vi "UserConsole.vi"(8 "error in (no error)":errorcluster) -> (0 "error out":errorcluster)   [LabVIEW 2013, in "UserConsole.lvlib"]
doc: "User Console simulates to Keypad,Transactions and Card Insertion."
uses:
  UserConsole.lvlib
  PrivateControls/Keypad.ctl
  PrivateControls/Transactions.ctl
  PrivateControls/UserConsole_QueueDriver.ctl
  MainVI/TopLevelController/ToplevelControllerLibrary.lvlib
panel:
  in  "Transactions":T1
  in  "Keypad":T2
  in  "Card Reader":bool
  # "User Console simulates to Keypad,Transactions and Card Insertion."
  # "[Covers: UI1]"
  # "[Covers: UI2C]"
  # "[Covers: UI2B]"
  # "[Covers: UI2]"
  # "[Covers: UI2A]"
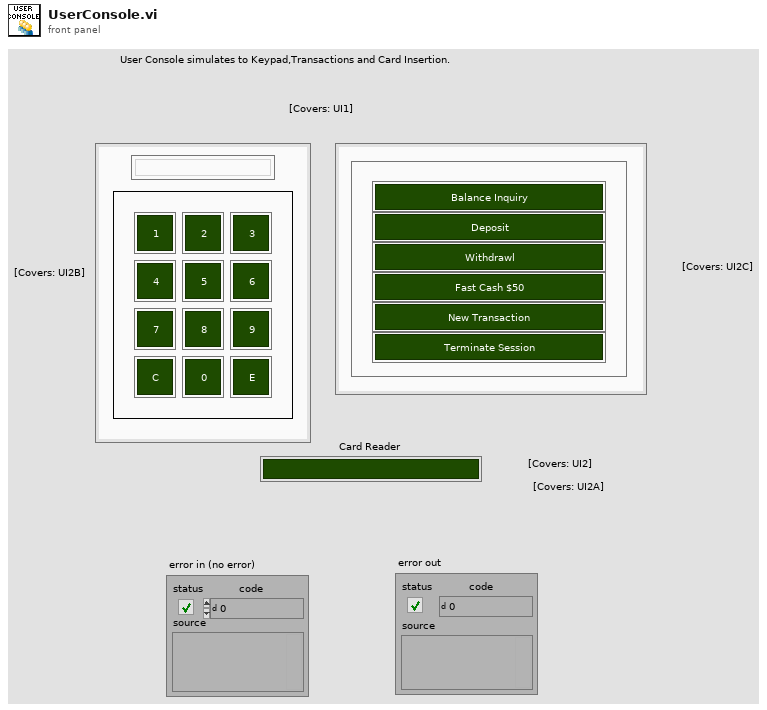
[diagram p1: front panel]
types:
  T1 = typedef "UserConsole.lvlib/Transactions.ctl" = cluster{"xaction":bool, "xaction 2":bool, "xaction 3":bool, "xaction 4":bool, "xaction 5":bool, "xaction 6":bool}
  T2 = typedef "UserConsole.lvlib/Keypad.ctl" = cluster{"Key":bool, "Key 2":bool, "Key 3":bool, "Key 4":bool, "Key 5":bool, "Key 6":bool, "Key 7":bool, "Key 8":bool, "Key 9":bool, "Key 10":bool, "Key 11":bool, "Key 12":bool, "Knumber":string}
  T3 = typedef "UserConsole.lvlib/UserConsole_QueueDriver.ctl" = enum16{"Default Case", "Init", "Enqueue", "Dequeue", "ReleaseQueue", "Exit"}
  T4 = enum16{"Create Event", "Generate Event", "Destroy Event"}
  T5 = enum16{"Init", "Enqueue", "Dequeue", "ReleaseQueue", "Exit"}
  T6 = typedef "UserConsole.lvlib/DataCluster.ctl" = cluster{"Card Reader":bool, "Keypad":cluster{"Key":bool, "Key 2":bool, "Key 3":bool, "Key 4":bool, "Key 5":bool, "Key 6":bool, "Key 7":bool, "Key 8":bool, "Key 9":bool, "Key 10":bool, "Key 11":bool, "Key 12":bool, "Knumber":string}, "Transactions":cluster{"xaction":bool, "xaction 2":bool, "xaction 3":bool, "xaction 4":bool, "xaction 5":bool, "xaction 6":bool}}
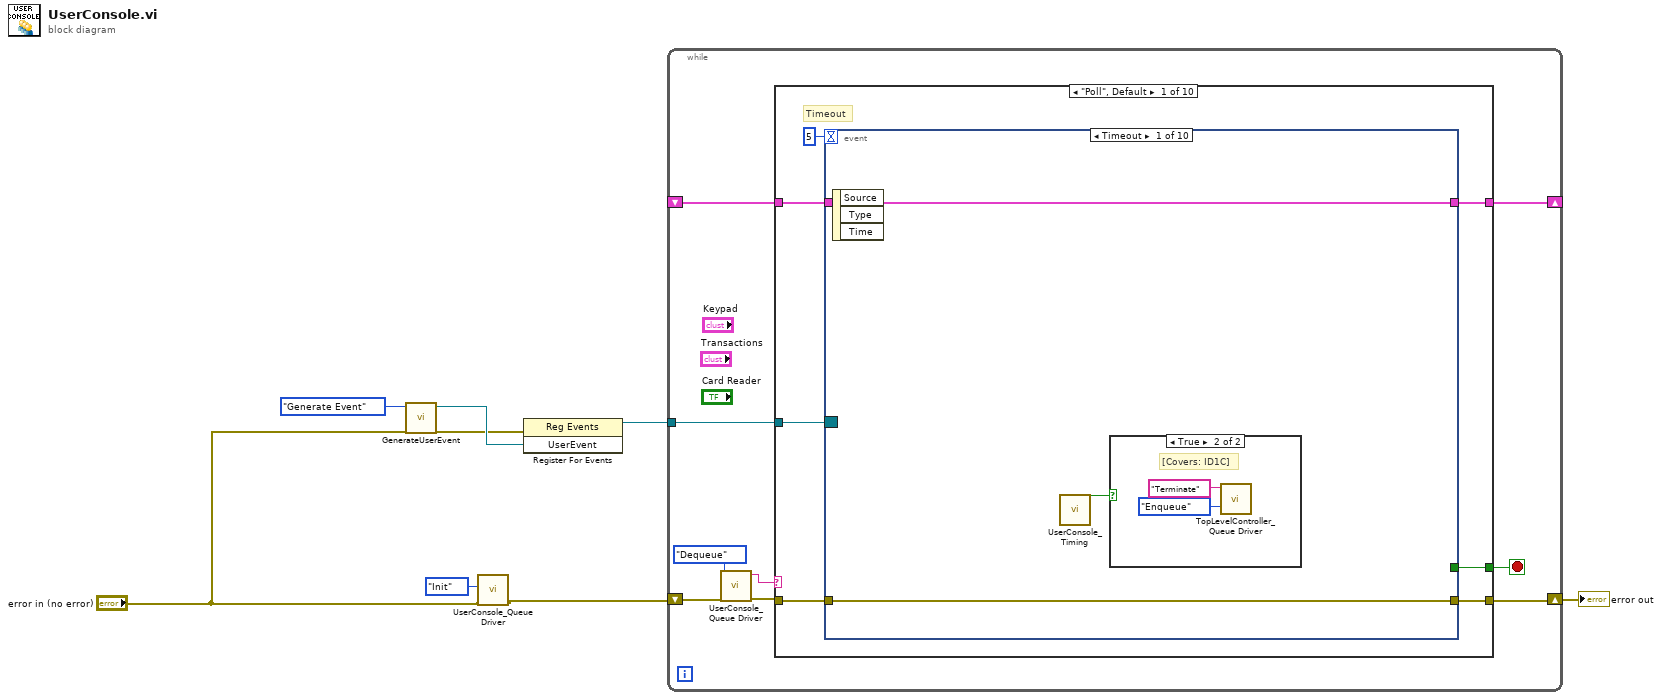
[diagram p0: block diagram]
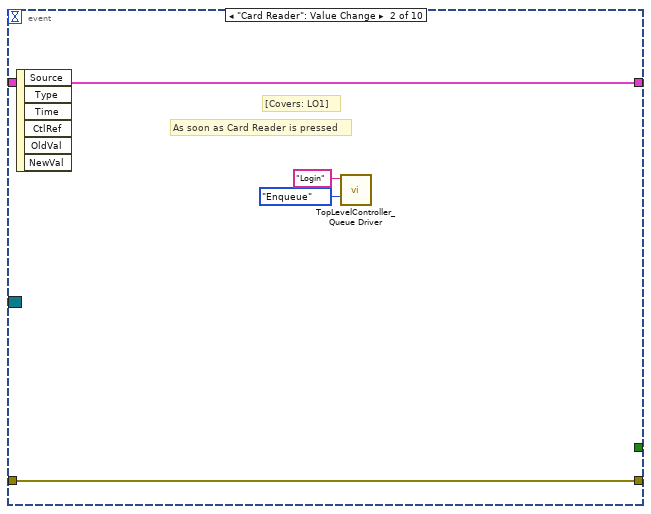
[diagram p3: hidden frame]
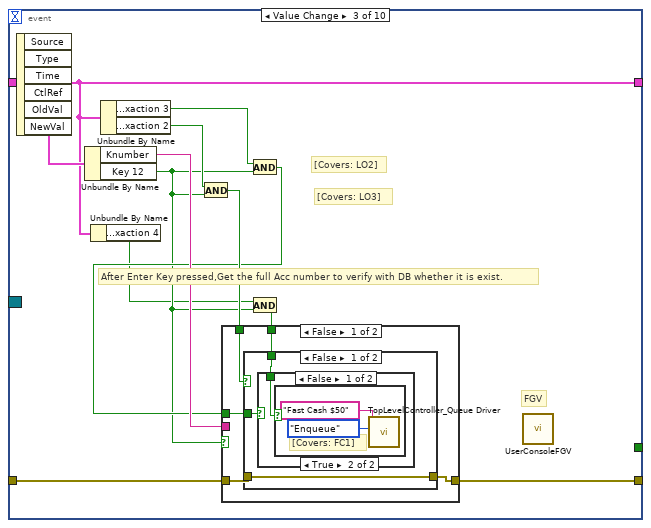
[diagram p4: hidden frame]
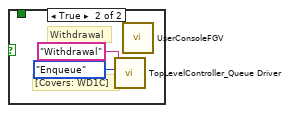
[diagram p6: hidden frame]
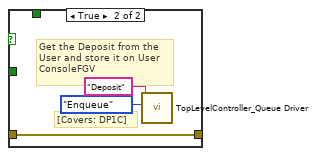
[diagram p7: hidden frame]
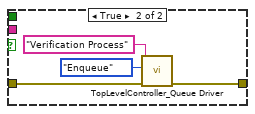
[diagram p8: hidden frame]
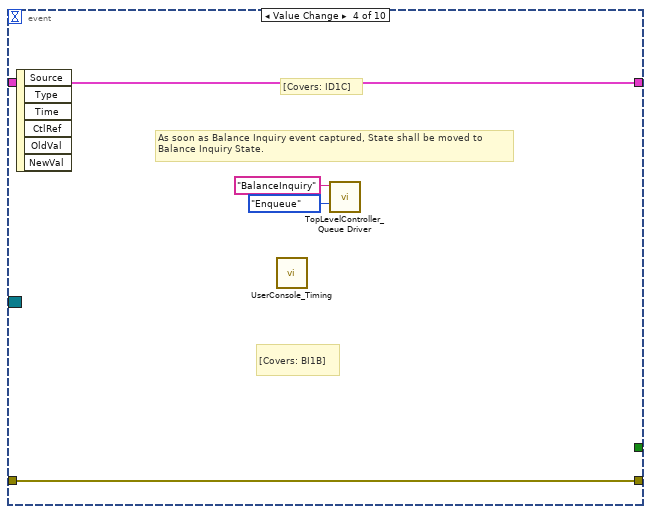
[diagram p9: hidden frame]
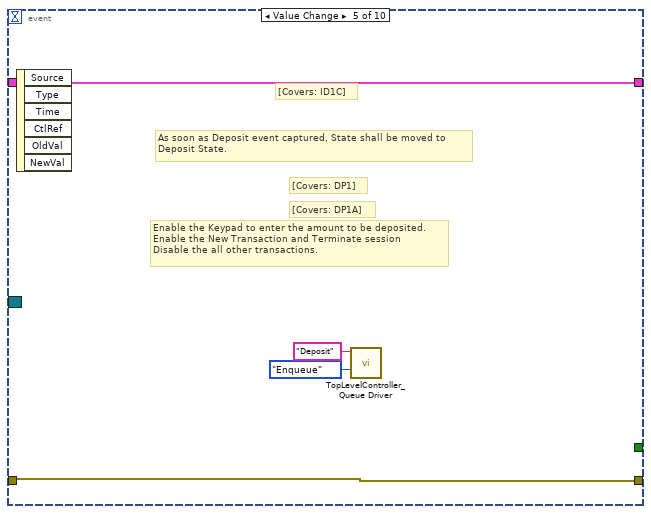
[diagram p10: hidden frame]
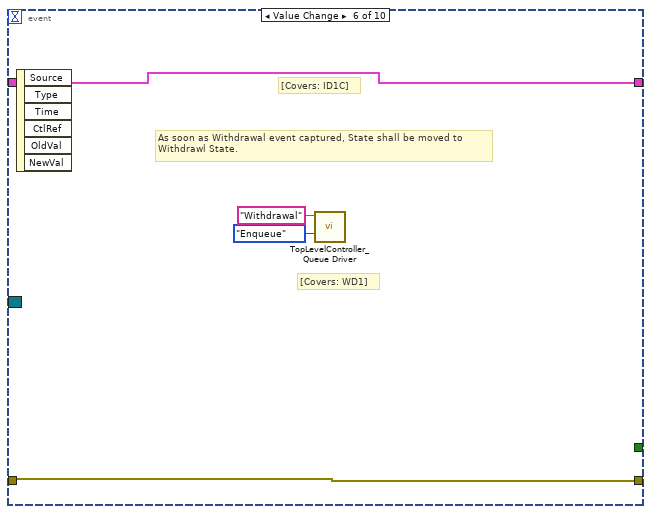
[diagram p11: hidden frame]
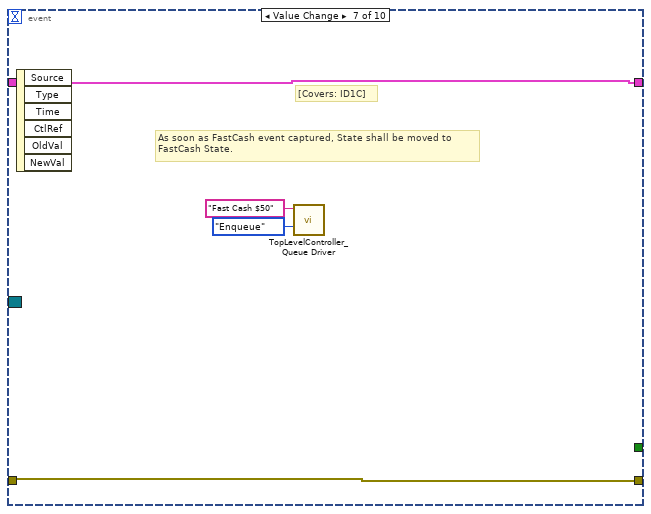
[diagram p12: hidden frame]
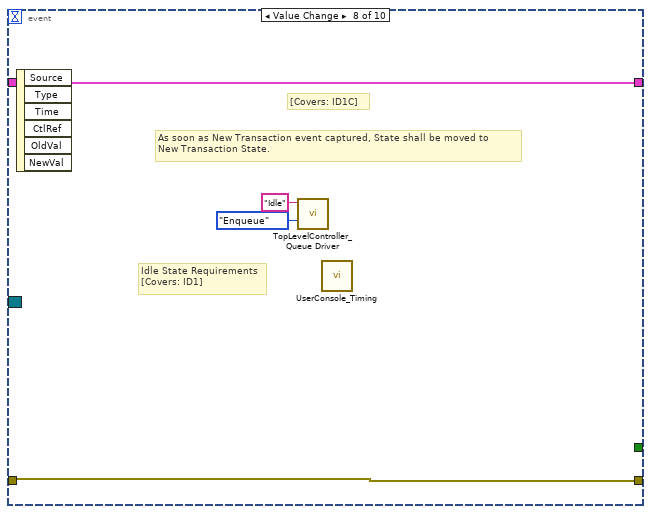
[diagram p13: hidden frame]
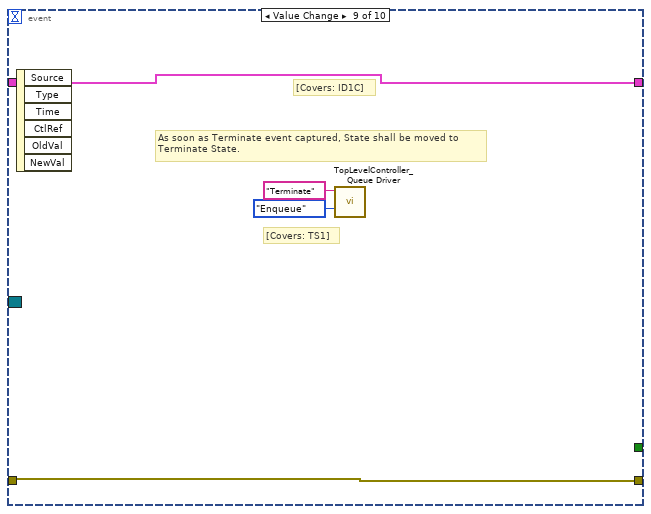
[diagram p14: hidden frame]
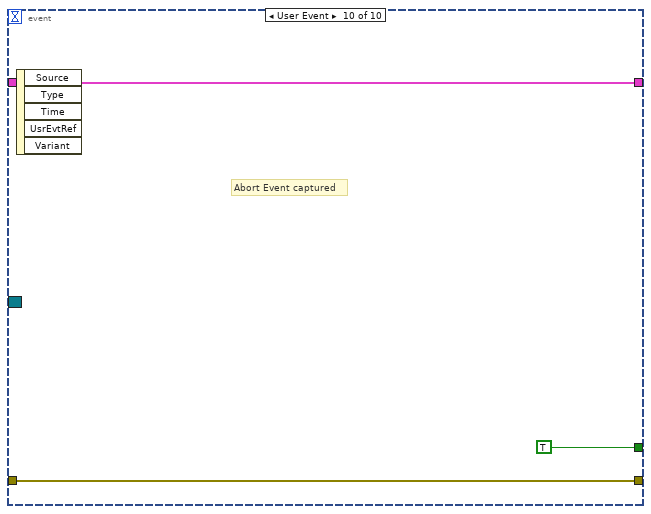
[diagram p15: hidden frame]
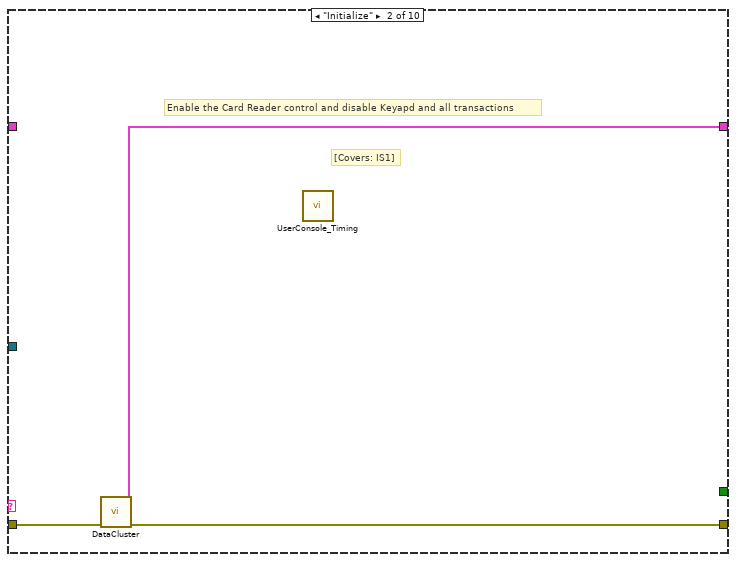
[diagram p16: hidden frame]
diagram:
  n1 = call "GenerateUserEvent.vi"("Event Actions"=T4."Generate Event") -> ("UserEvent"=w4:refnum<user-event>)  [unwired: 9 in, 1 out]
  n2 = call "UserConsole_Queue Driver.vi"("error in (no error)"="error in (no error)", "State"=UserConsole_QueueDriver."Init") -> ("error out"=w3:errorcluster)  [unwired: 8 in, 1 out]
  n3 = register-events(error in="error in (no error)", w4) -> (reference out=w6:refnum<event-registration>)  [unwired: 1 in, 1 out]
  n4 = while {
    shift-right: [w16] -> w7
    shift-left: w3 -> [w11]
    tunnel: w6 -> [w15]
    shift-right: [w12] -> _
    shift-left: _ -> [w13]
    stop <- w14 stop-if-true
    n5 = call "UserConsole_Queue Driver.vi"("error in (no error)"=w11, "State"=UserConsole_QueueDriver."Dequeue") -> ("error out"=w10:errorcluster, "DeQ"=w9:string)  [unwired: 8 in]
    n6 = case shown="\"Poll\", Default" w9 {
      tunnel: w10 -> [w23 w94 w96 w98 w99 w101 w104 w105 w110 w112]
      tunnel: [w22 w93 w96 w98 w99 w101 w104 w105 w110 w112] -> w16
      tunnel: w15 -> [w21 _ _ _ _ _ _ _ _ _]
      tunnel: [w20 _ _ _ _ _ _ _ _ _] -> w14
      tunnel: w13 -> [w18 _ w95 w97 w100 w102 w103 w106 w109 w111]
      tunnel: [w17 w92 w95 w97 w100 w102 w103 w106 w109 w111] -> w12
      frame "Poll", Default {
        # "Timeout"
        n7 = event shown="[0] Timeout" {
          selector: w21 -> [_ _ _ _ _ _ _ _ _ _]
          dyn-events: _ -> [_ _ _ _ _ _ _ _ _ _]
          timeout: 5 -> [_ _ _ _ _ _ _ _ _ _]
          tunnel: w23 -> [w26 w31 w43 w68 w72 w75 w79 w84 w87 w89]
          tunnel: [w26 w31 w42 w68 w72 w75 w79 w84 w87 w89] -> w22
          tunnel: [_ _ _ _ _ _ _ _ _ TRUE] -> w20
          tunnel: w18 -> [w25 w32 w33 w65 w69 w76 w80 w83 w88 w90]
          tunnel: [w25 w32 w33 w65 w69 w76 w80 w83 w88 w90] -> w17
          event Timeout {
            n8 = event-data() -> ()  [unwired: 1 in, 3 out]
            n9 = call "UserConsole_Timing.vi"() -> ("Elapsed?"=w24:bool)  [unwired: 11 in]
            n10 = case shown="True" w24 {
              frame False {
              }
              frame True {
                # "[Covers: ID1C]"
                n11 = call "TopLevelController_Queue Driver.vi"("Enum"=T5."Enqueue", "EnQ"="Terminate") -> ()  [unwired: 8 in, 2 out]
              }
            }
          }
          event "Card Reader": Value Change {
            # "[Covers: LO1]"
            # "As soon as Card Reader is pressed"
            n12 = event-data() -> ()  [unwired: 1 in, 6 out]
            n13 = call "TopLevelController_Queue Driver.vi"("Enum"=T5."Enqueue", "EnQ"="Login") -> ()  [unwired: 8 in, 2 out]
          }
          event Value Change {
            # "FGV"
            # "[Covers: LO3]"
            # "[Covers: LO2]"
            # "After Enter Key pressed,Get the full Acc number to verify with DB whether it is exist."
            n14 = event-data() -> ("NewVal"=w44:T2)  [unwired: 1 in, 5 out]
            n15 = Unbundle By Name(w44) -> ("Knumber"=w41:string, "Key 12"=w35:bool)
            n16 = Unbundle By Name(w33) -> ("Transactions.xaction 4"=w34:bool)
            n17 = Unbundle By Name(w33) -> ("Transactions.xaction 3"=w38:bool, "Transactions.xaction 2"=w40:bool)
            n18 = And(x=w40, y=w35) -> (x .and. y?=w39:bool)
            n19 = And(x=w38, y=w35) -> (x .and. y?=w37:bool)
            n20 = And(x=w34, y=w35) -> (x .and. y?=w36:bool)
            n21 = case shown="False" w35 {
              tunnel: w43 -> [w48 w62]
              tunnel: [w47 w61] -> w42
              tunnel: w41 -> [_ _]
              tunnel: w39 -> [w49 _]
              tunnel: w37 -> [w46 _]
              tunnel: w36 -> [w45 _]
              frame False {
                n22 = case shown="False" w49 {
                  tunnel: w48 -> [w52 w60]
                  tunnel: [w52 w60] -> w47
                  tunnel: w46 -> [w51 _]
                  tunnel: w45 -> [w50 _]
                  frame False {
                    n23 = case shown="False" w51 {
                      tunnel: w50 -> [w53 _]
                      frame False {
                        n24 = case shown="True" w53 {
                          frame False {
                          }
                          frame True {
                            # "[Covers: FC1]"
                            n25 = call "TopLevelController_Queue Driver.vi"("Enum"=T5."Enqueue", "EnQ"="Fast Cash $50") -> ()  [unwired: 8 in, 2 out]
                          }
                        }
                      }
                      frame True {
                        # "[Covers: WD1C]"
                        # "Withdrawal"
                        n26 = call "TopLevelController_Queue Driver.vi"("Enum"=T5."Enqueue", "EnQ"="Withdrawal") -> ()  [unwired: 8 in, 2 out]
                        n27 = call "UserConsoleFGV.vi"() -> ()  [unwired: 10 in, 2 out]
                      }
                    }
                  }
                  frame True {
                    # "Get the Deposit from the \nUser and store it on User\nConsoleFGV"
                    # "[Covers: DP1C]"
                    n28 = call "TopLevelController_Queue Driver.vi"("Enum"=T5."Enqueue", "EnQ"="Deposit") -> ()  [unwired: 8 in, 2 out]
                  }
                }
              }
              frame True {
                n29 = call "TopLevelController_Queue Driver.vi"("error in (no error)"=w62, "Enum"=T5."Enqueue", "EnQ"="Verification Process") -> ("error out"=w61:errorcluster)  [unwired: 7 in, 1 out]
              }
            }
            n30 = call "UserConsoleFGV.vi"() -> ()  [unwired: 10 in, 2 out]
          }
          event Value Change {
            # "[Covers: BI1B]"
            # "[Covers: ID1C]"
            # "As soon as Balance Inquiry event captured, State shall be moved to \nBalance Inquiry State."
            n31 = event-data() -> ()  [unwired: 1 in, 6 out]
            n32 = call "UserConsole_Timing.vi"() -> ()  [unwired: 11 in, 1 out]
            n33 = call "TopLevelController_Queue Driver.vi"("Enum"=T5."Enqueue", "EnQ"="BalanceInquiry") -> ()  [unwired: 8 in, 2 out]
          }
          event Value Change {
            # "[Covers: DP1A]"
            # "Enable the Keypad to enter the amount to be deposited.\nEnable the New Transaction and Terminate session \nDisable the all other transactions."
            # "[Covers: DP1]"
            # "[Covers: ID1C]"
            # "As soon as Deposit event captured, State shall be moved to \nDeposit State."
            n34 = event-data() -> ()  [unwired: 1 in, 6 out]
            n35 = call "TopLevelController_Queue Driver.vi"("Enum"=T5."Enqueue", "EnQ"="Deposit") -> ()  [unwired: 8 in, 2 out]
          }
          event Value Change {
            # "[Covers: WD1]"
            # "[Covers: ID1C]"
            # "As soon as Withdrawal event captured, State shall be moved to \nWithdrawl State."
            n36 = event-data() -> ()  [unwired: 1 in, 6 out]
            n37 = call "TopLevelController_Queue Driver.vi"("Enum"=T5."Enqueue", "EnQ"="Withdrawal") -> ()  [unwired: 8 in, 2 out]
          }
          event Value Change {
            # "[Covers: ID1C]"
            # "As soon as FastCash event captured, State shall be moved to \nFastCash State."
            n38 = event-data() -> ()  [unwired: 1 in, 6 out]
            n39 = call "TopLevelController_Queue Driver.vi"("Enum"=T5."Enqueue", "EnQ"="Fast Cash $50") -> ()  [unwired: 8 in, 2 out]
          }
          event Value Change {
            # "Idle State Requirements\n[Covers: ID1]"
            # "[Covers: ID1C]"
            # "As soon as New Transaction event captured, State shall be moved to \nNew Transaction State."
            n40 = event-data() -> ()  [unwired: 1 in, 6 out]
            n41 = call "TopLevelController_Queue Driver.vi"("Enum"=T5."Enqueue", "EnQ"="Idle") -> ()  [unwired: 8 in, 2 out]
            n42 = call "UserConsole_Timing.vi"() -> ()  [unwired: 11 in, 1 out]
          }
          event Value Change {
            # "[Covers: TS1]"
            # "[Covers: ID1C]"
            # "As soon as Terminate event captured, State shall be moved to \nTerminate State."
            n43 = event-data() -> ()  [unwired: 1 in, 6 out]
            n44 = call "TopLevelController_Queue Driver.vi"("Enum"=T5."Enqueue", "EnQ"="Terminate") -> ()  [unwired: 8 in, 2 out]
          }
          event User Event {
            # "Abort Event captured"
            n45 = event-data() -> ()  [unwired: 1 in, 5 out]
          }
        }
      }
      frame "Initialize" {
        # "[Covers: IS1]"
        # "Enable the Card Reader control and disable Keyapd and all transactions"
        n46 = call "DataCluster.vi"("error in (no error)"=w94) -> ("error out"=w93:errorcluster, "Data Cluster"=w92:T6)  [unwired: 9 in]
        n47 = call "UserConsole_Timing.vi"() -> ()  [unwired: 11 in, 1 out]
      }
      frame "Idle" {
        # "[Covers: ID1A]"
        # "Disable the Keypad and Enable the All Transactions"
        # "Turn ON the Card Reader and disable the same"
      }
      frame "Login" {
        # "[Covers: LO1A]"
        # "Keep Card Reader ON and disabled.\nEnable the Keypad and Terminate Session\nDisable the All other transactions."
      }
      frame "Deposit" {
        # "[Covers: DP1A]"
        # "Disable all other transactions"
        # "Enable the Keypad , New Transaction and Terminate Session"
      }
      frame "Withdrawal" {
        # "[Covers: WD1A]"
        # "Disable all other transactions"
        # "Enable the Keypad , New Transaction and Terminate Session"
      }
      frame "Fast Cash $50" {
        # "[Covers: FC1A]"
        # "Disable all transactions"
        # "Enable the New Transaction and Terminate session"
      }
      frame "Terminate" {
        # "[Covers: TS1A]"
        # "Disable all user controls"
      }
      frame "Error" {
        # "Once Error occured, Error info will be moved to Centralized Error handler"
        n48 = call "TopLevelController_Queue Driver.vi"("Enum"=T5."Enqueue", "EnQ"="Error") -> ()  [unwired: 8 in, 2 out]
      }
      frame "Exit" {
      }
    }
  }
  "error out" <- w7
